vi "ZMC Search And Open Com.vi"(6 "phandle":u32, 7 "uims":u32, 8 "error in (no error)":errorcluster caption="错误输入（无错误）", 9 "pcomid":u32, 10 "uimaxcomidfind":u32, 11 "uimincomidfind":u32) -> (0 "error out":errorcluster caption="错误输出", 1 "pcomid out":u32, 3 "function return":i32, 4 "phandle out":u32)   [LabVIEW 2015, in "zauxdll.lvlib"]
doc: "int32 __stdcall ZMC_SearchAndOpenCom(uint32 uimincomidfind, uint32 uimaxcomidfind,uint* pcomid, uint32 uims, ZMC_HANDLE * phandle);"
uses:
  zauxdll.lvlib
  zmotion.dll
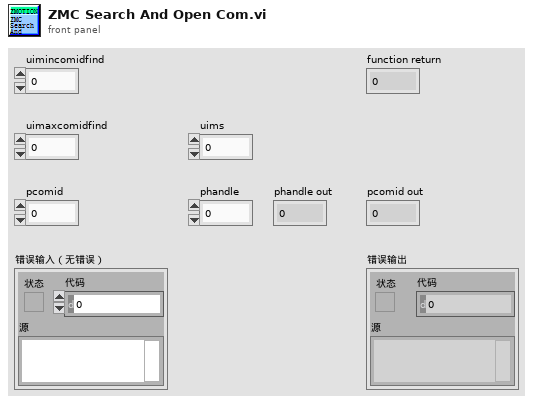
[diagram p1: front panel]
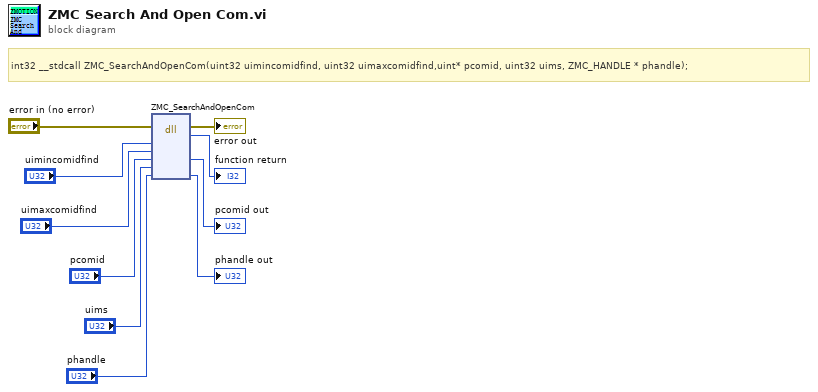
[diagram p0: block diagram]
diagram:
  # "int32 __stdcall ZMC_SearchAndOpenCom(uint32 uimincomidfind, uint32 uimaxcomidfind,uint* pcomid, uint32 uims, ZMC_HANDLE * phandle);"
  n1 = dll-call lib="C:/Users/VIC/Desktop/GOGORO_SA/system/LLB/zmotion/zaux/zmotion.*" fn="ZMC_SearchAndOpenCom"(error in="error in (no error)", "uimincomidfind"="uimincomidfind", "uimaxcomidfind"="uimaxcomidfind", "pcomid"="pcomid", "uims"="uims", "phandle"="phandle") -> (error out=→"error out":errorcluster, →"function return":i32, "pcomid"=→"pcomid out":u32, "phandle"=→"phandle out":u32)  [unwired: 5 in, 1 out]
